vi "Get LR700 data_VISA.vi"(4 "error in (no error)":errorcluster, 5 "Data chanel":enum16{"R", "X"}(ring), 6 "Max repetitions":i32=6, 7 "VISA resource name":refnum<visa-resource-name>) -> (0 "error out":errorcluster, 2 "Data":dbl format="%.4e", 3 "VISA resource name out":refnum<visa-resource-name>)   [LabVIEW 2019]
uses:
  GPIB/VISA  Send Receive.vi
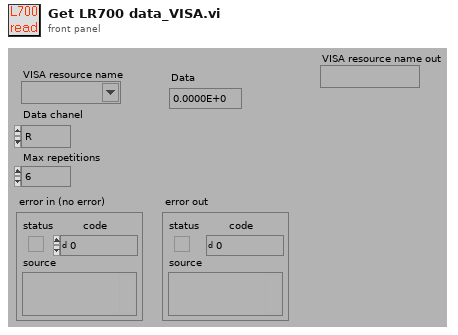
[diagram p1: front panel]
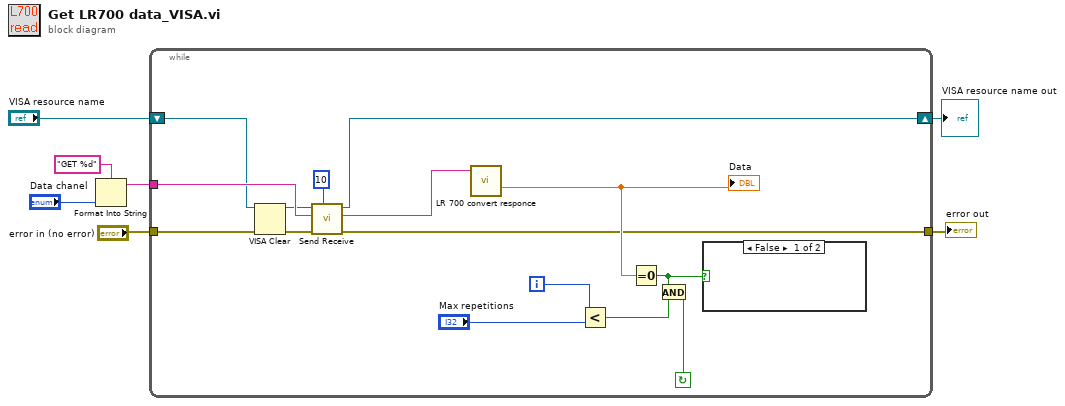
[diagram p0: block diagram]
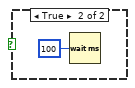
[diagram p2: hidden frame]
diagram:
  n1 = Format Into String(format string="GET %d", "Data chanel") -> (resulting string=w5:string)  [unwired: 2 in, 1 out]
  n2 = while {
    tunnel: [w11] -> w3
    tunnel: "error in (no error)" -> [w12]
    tunnel: w5 -> [w16]
    shift-right: [w8] -> w1
    shift-left: "VISA resource name" -> [w10]
    i -> [w21]
    stop <- w18 continue-if-true
    n3 = VISA Clear(VISA resource name=w10, error in (no error)=w12) -> (VISA resource name out=w9:refnum<visa-resource-name>, error out=w15:errorcluster)
    n4 = call-poly "Send Receive.vi"("Read Delay, ms"=u32 10 ("Delay, ms"), "error in (no error)"=w15, "data string in"=w16, "VISA Resource Name"=w9) -> ("error out"=w11:errorcluster, "data string out"=w13:string, "VISA Resource Name Out"=w8:refnum<visa-resource-name>)  [unwired: 5 in]
    n5 = call "LR 700 convert responce.vi"("LR 700 Responce"=w13) -> ("Resistance"=w22:dbl)  [unwired: 2 out]
    "Data" <- w22
    n6 = Less?(x=w21, y="Max repetitions") -> (x < y?=w19:bool)
    n7 = Equal To 0?(x=w22) -> (x = 0?=w17:bool)
    n8 = And(x=w17, y=w19) -> (x .and. y?=w18:bool)
    n9 = case shown="False" w17 {
      frame False {
      }
      frame True {
        n10 = Wait (ms)(milliseconds to wait=u32 100) -> ()  [unwired: 1 out]
      }
    }
  }
  "error out" <- w3
  "VISA resource name out" <- w1
